vi "OPC Read.vi"(8 "error in (no error)":errorcluster, 9 "OPCServer_Location":string, 10 "Mode":T1=enum."Initialize") -> (0 "error out":errorcluster, 1 "Time out from server":bool, 2 "Value":bool, 3 "data":i32, 5 "date":string)   [LabVIEW 2019]
doc: "This VI reads multiple OPC items at one time. Specify which items you want to read or use the predetermined list of items. The predetermined list of items specifies items from the National Instruments.OPCDemo server, which has been installed on your machine."
uses:
  Read Mode.ctl
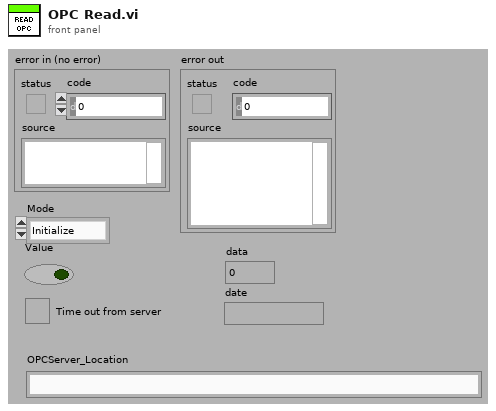
[diagram p1: front panel]
types:
  T1 = typedef "Read Mode.ctl" = enum16{"PLC_to_PC", "Partnumber_to_PC", "Initialize", "Close"}
  T2 = enum16{"Read", "Write", "ReadWrite", "BufferedRead", "BufferedReadWrite"}
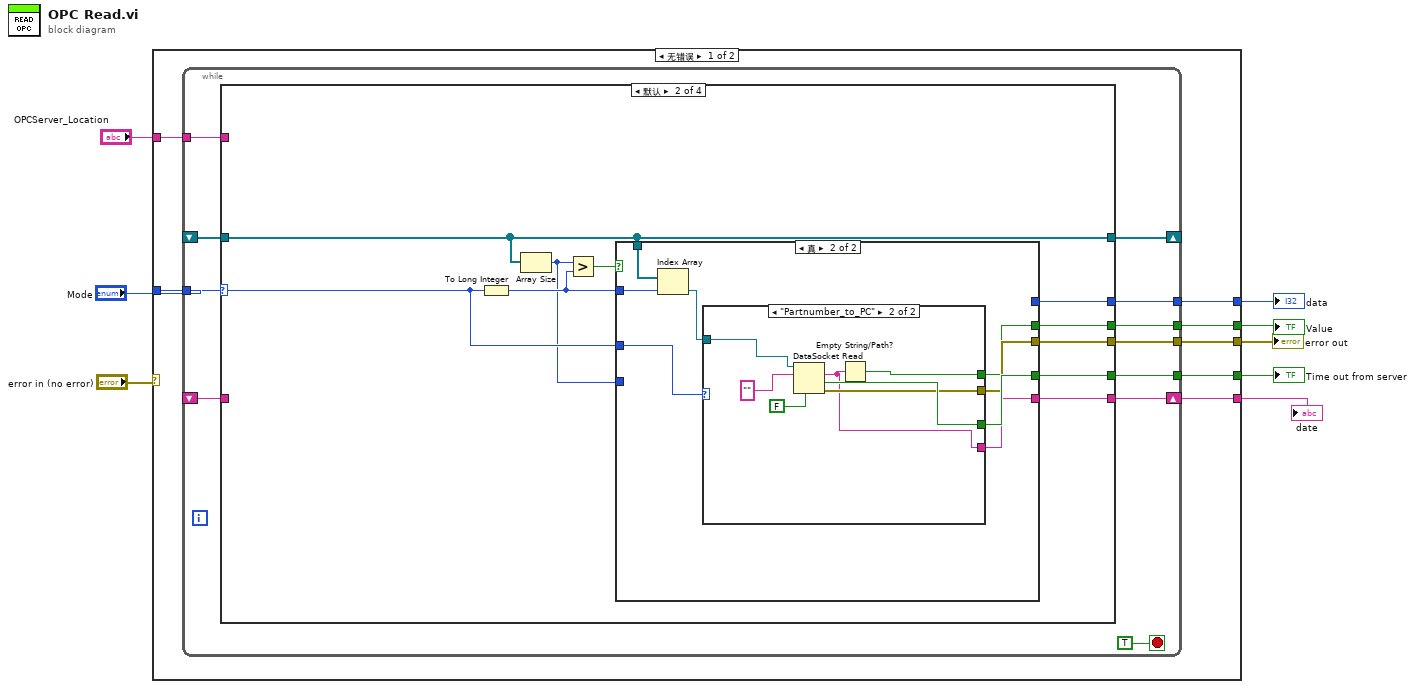
[diagram p0: block diagram]
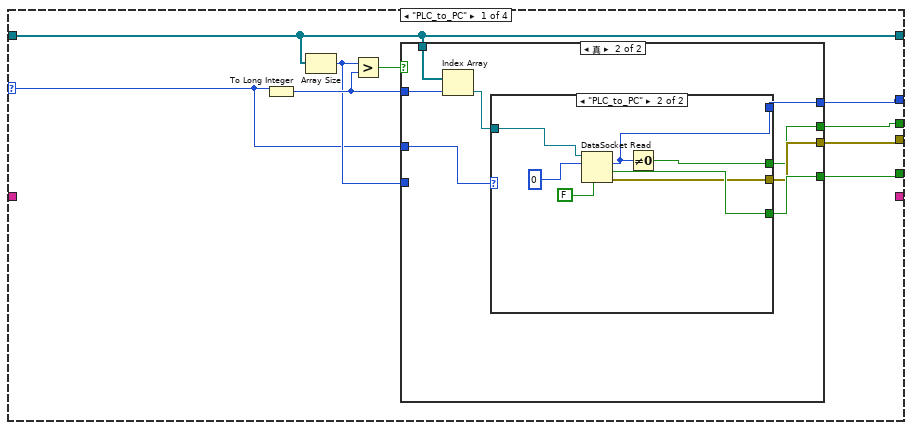
[diagram p2: hidden frame]
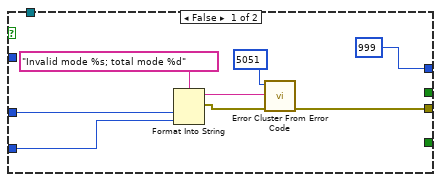
[diagram p3: hidden frame]
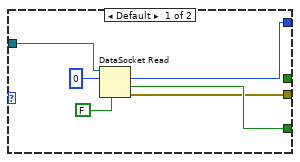
[diagram p4: hidden frame]
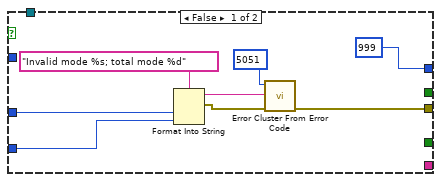
[diagram p5: hidden frame]
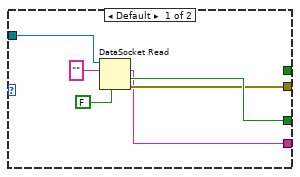
[diagram p6: hidden frame]
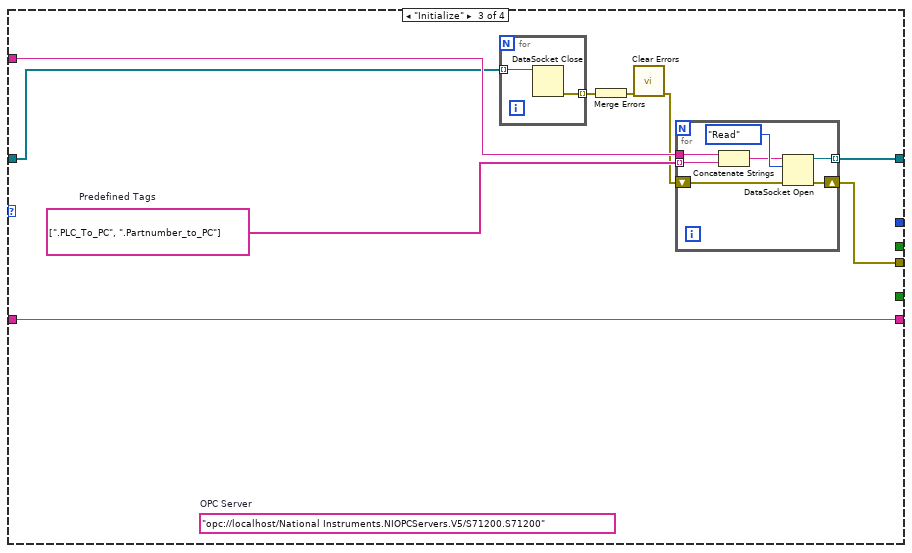
[diagram p7: hidden frame]
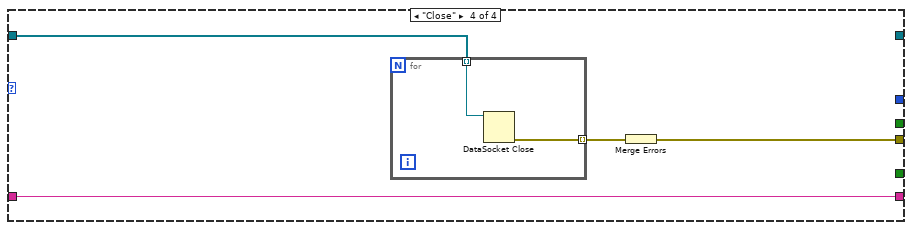
[diagram p8: hidden frame]
diagram:
  n1 = case shown="无错误" "error in (no error)" {
    selector: "error in (no error)" -> [_ w128]
    tunnel: "Mode" -> [w15 _]
    tunnel: [w14 w128] -> w7
    tunnel: [w13 _] -> w6
    tunnel: [w12 _] -> w4
    tunnel: [w11 _] -> w3
    tunnel: "OPCServer_Location" -> [w10 _]
    tunnel: [w9 _] -> w1
    frame No Error {
      n2 = while {
        shift-right: [w25] -> _
        shift-left: _ -> [w22]
        tunnel: w15 -> [w24]
        tunnel: [w23] -> w14
        tunnel: [w21] -> w13
        tunnel: [w20] -> w12
        tunnel: [w19] -> w11
        tunnel: w10 -> [w18]
        shift-right: [w17] -> w9
        shift-left: _ -> [w16]
        stop <- TRUE stop-if-true
        n3 = case shown="默认" w24 {
          selector: w24 -> [w31 w67 _ _]
          tunnel: [w32 w70 w111 _] -> w25
          tunnel: [w29 w73 w106 w123] -> w23
          tunnel: w22 -> [w32 w70 w109 w125]
          tunnel: [w30 w74 _ _] -> w21
          tunnel: [w28 w72 _ _] -> w20
          tunnel: [w27 w71 _ _] -> w19
          tunnel: w18 -> [_ _ w110 _]
          tunnel: [_ w65 w104 w122] -> w17
          tunnel: w16 -> [_ _ w104 w122]
          frame "PLC_to_PC" {
            n4 = To Long Integer(number=w31) -> (32bit integer=w35:i32)
            n5 = Array Size(array=w32) -> (size(s)=w33:i32)
            n6 = Greater?(x=w33, y=w35) -> (0:w34:bool)
            n7 = case shown="真" w34 {
              tunnel: [_ w50] -> w30
              tunnel: [w43 w49] -> w29
              tunnel: [_ w48] -> w28
              tunnel: [999 w45] -> w27
              tunnel: w32 -> [_ w47]
              tunnel: w35 -> [_ w44]
              tunnel: w31 -> [w41 w46]
              tunnel: w33 -> [w37 _]
              frame False {
                n8 = Format Into String(format string="Invalid mode %s; total mode %d" ("error message (\"\")"), w41, w37) -> (resulting string=w39:string, error out=w38:errorcluster)  [unwired: 2 in]
                n9 = call <vilib>:"Error Cluster From Error Code.vi"("error in (no error)"=w38, "error message (\"\")"=w39, "error code (0)"=5051) -> ("error out"=w43:errorcluster)  [unwired: 6 in]
              }
              frame True {
                n10 = Index Array(array=w47, index=w44) -> (element=w51:refnum<k13>)
                n11 = case shown="\"PLC_to_PC\"" w46 {
                  tunnel: w51 -> [w56 w59]
                  tunnel: [w55 w63] -> w50
                  tunnel: [w54 w62] -> w49
                  tunnel: [_ w61] -> w48
                  tunnel: [w52 w58] -> w45
                  frame Default {
                    n12 = DataSocket Read(6:FALSE ("wait for updated value (T)"), 10:0, 11:w56) -> (0:w54:errorcluster, 1:w55:bool, 2:w52:i32)  [unwired: 2 in, 4 out]
                  }
                  frame "PLC_to_PC" {
                    n13 = DataSocket Read(6:FALSE ("wait for updated value (T)"), 10:0, 11:w59) -> (0:w62:errorcluster, 1:w63:bool, 2:w58:i32)  [unwired: 2 in, 4 out]
                    n14 = Not Equal To 0?(x=w58) -> (x != 0?=w61:bool)
                  }
                }
              }
            }
          }
          frame Default {
            n15 = To Long Integer(number=w67) -> (32bit integer=w69:i32)
            n16 = Array Size(array=w70) -> (size(s)=w66:i32)
            n17 = Greater?(x=w66, y=w69) -> (0:w68:bool)
            n18 = case shown="真" w68 {
              tunnel: [_ w89] -> w74
              tunnel: [w82 w88] -> w73
              tunnel: [_ w87] -> w72
              tunnel: [999 _] -> w71
              tunnel: w70 -> [_ w86]
              tunnel: w69 -> [_ w83]
              tunnel: w67 -> [w80 w85]
              tunnel: w66 -> [w76 _]
              tunnel: [_ w84] -> w65
              frame False {
                n19 = Format Into String(format string="Invalid mode %s; total mode %d" ("error message (\"\")"), w80, w76) -> (resulting string=w78:string, error out=w77:errorcluster)  [unwired: 2 in]
                n20 = call <vilib>:"Error Cluster From Error Code.vi"("error in (no error)"=w77, "error message (\"\")"=w78, "error code (0)"=5051) -> ("error out"=w82:errorcluster)  [unwired: 6 in]
              }
              frame True {
                n21 = Index Array(array=w86, index=w83) -> (element=w90:refnum<k13>)
                n22 = case shown="\"Partnumber_to_PC\"" w85 {
                  tunnel: w90 -> [w95 w97]
                  tunnel: [w94 w102] -> w89
                  tunnel: [w93 w101] -> w88
                  tunnel: [_ w100] -> w87
                  tunnel: [w91 w99] -> w84
                  frame Default {
                    n23 = DataSocket Read(6:FALSE ("wait for updated value (T)"), 10:"", 11:w95) -> (0:w93:errorcluster, 1:w94:bool, 2:w91:string)  [unwired: 2 in, 4 out]
                  }
                  frame "Partnumber_to_PC" {
                    n24 = DataSocket Read(6:FALSE ("wait for updated value (T)"), 10:"", 11:w97) -> (0:w101:errorcluster, 1:w102:bool, 2:w99:string)  [unwired: 2 in, 4 out]
                    n25 = Empty String/Path?(string/path=w99) -> (empty?=w100:bool)
                  }
                }
              }
            }
          }
          frame "Initialize" {
            (unwired) "opc://localhost/National Instruments.NIOPCServers.V5/S71200.S71200"  # OPC Server
            w112 = string[] [".PLC_To_PC", ".Partnumber_to_PC"]  # Predefined Tags
            n26 = for {
              tunnel: w109 -> [w114] mode=indexing
              tunnel: [w113] -> w108 mode=indexing
              n27 = DataSocket Close(11:w114) -> (0:w113:errorcluster)  [unwired: 2 in, 1 out]
            }
            n28 = Merge Errors(w108) -> (w107:errorcluster)
            n29 = call <vilib>:"Clear Errors.vi"("error in (no error)"=w107) -> ("error out"=w105:errorcluster)  [unwired: 5 in, 1 out]
            n30 = for {
              tunnel: w112 -> [w116] mode=indexing
              tunnel: w110 -> [w117]
              tunnel: [w119] -> w111 mode=indexing
              shift-right: [w118] -> w106
              shift-left: w105 -> [w115]
              n31 = Concatenate Strings(w117, w116) -> (w120:string)
              n32 = DataSocket Open(8:w115, 10:T2."Read" ("mode"), 11:w120) -> (0:w118:errorcluster, 3:w119:refnum<k13>)  [unwired: 1 out]
            }
          }
          frame "Close" {
            n33 = for {
              tunnel: [w127] -> w124 mode=indexing
              tunnel: w125 -> [w126] mode=indexing
              n34 = DataSocket Close(11:w126) -> (0:w127:errorcluster)  [unwired: 2 in, 1 out]
            }
            n35 = Merge Errors(w124) -> (w123:errorcluster)
          }
        }
      }
    }
    frame Error {
    }
  }
  "Value" <- w4
  "error out" <- w7
  "Time out from server" <- w6
  "data" <- w3
  "date" <- w1
